vi "_LOharmonic.vi"(0 "Bias_LO_equip":T5={"Node address"=19, "CAN Interface"="CAN0", "Cartridge band"=10, "Slave Node in"={"Address"=19, "Serial Number"=[16, -88, -112, 75, 1, 8, 0, 24]}, "ObjHandle out"=19, "POL"=0, "sb"=1, "GPIB_SM (SIS S,V)"="24", "GPIB_DMM (SIS I)"="22", "GPIB_SM (MAG I) "="25", "GPIB_SG(LO)"="19", "GPIB_PW (PAMP) "="6", "GPIB_TMP1(8ch)"="12", "GPIB_TMP2(2ch)  "="13", "WCA_avg"=10, "Rsen"=10.0, "BiasModule"=1, "LOModule "=2, "WCA_LO_FREQ_SET"={"YTO Low freq. [GHz]"=14.66, "YTO High freq. [GHz]"=17.5, "Kvco"=1, "Lock Pol."=0, "SET LO FREQ"=88.77778, "Multiplier"=6.0, "YTO (HEX)"=197, "YTO ( FREQ)"=14.796625, "NULL PLL INTEGRATOR"=FALSE}, "Res for"=0} {"Res for" items=["none", "series res", "parallel res"]; "WCA_LO_FREQ_SET"."YTO ( FREQ)" min=25 max=150 step=0.0001 format="%.3f"; "WCA_LO_FREQ_SET"."Multiplier" min=3 max=6 step=3; "WCA_LO_FREQ_SET"."SET LO FREQ" min=25 max=150 step=0.0001 format="%.3f"; "WCA_LO_FREQ_SET"."Lock Pol." items=["Lower", "Upper"]; "WCA_LO_FREQ_SET"."Kvco" items=["7.5MHz/V", "15MHz/V"]; "WCA_LO_FREQ_SET"."YTO High freq. [GHz]" format="%.3f"; "WCA_LO_FREQ_SET"."YTO Low freq. [GHz]" format="%.3f"; "LOModule" items=["Manual Gunn+PAMP"=0, "PLL GUNN+PAMP"=5, "B10Lab LO"=1, "WCA LO"=2, ""=3, "YIG発信器"=4, "none"=99]; "BiasModule" items=["B10Lab Bias"=0, "WCA BiasModule"=1, "none"=99]; "Slave Node in"."Serial Number" format="%.0x"; "Slave Node in"."Address" format="%.0x"; "Cartridge band" max=10 step=1; "Node address" format="%.0x"}, 1 "Control":T9={"GPIB_ATT"="28", "6501Dev#"=1, "GPIB_SP"="18", "GPIB_PM"="13", "GPIB_DSA"="11", "GPIB_DMM (TPD)"="23", "GPIB_MPI"="COM3", "mortor設定"=[{"Axis"=0, "ID"=0, "HIspeed"=200.0, "LOspeed"=100.0, "ACCEL(ms)"=100.0, "Sratio"=50.0, "フリーラン\n"=FALSE, "文字列"="DSB HOT/COLD"}, {"Axis"=1, "ID"=0, "HIspeed"=4.0, "LOspeed"=4.0, "ACCEL(ms)"=100.0, "Sratio"=50.0, "フリーラン\n"=TRUE, "文字列"="SubMM Att"}, {"Axis"=0, "ID"=0, "HIspeed"=200.0, "LOspeed"=100.0, "ACCEL(ms)"=100.0, "Sratio"=50.0, "フリーラン\n"=FALSE, "文字列"="MPI Port1"}, {"Axis"=1, "ID"=0, "HIspeed"=200.0, "LOspeed"=100.0, "ACCEL(ms)"=100.0, "Sratio"=50.0, "フリーラン\n"=FALSE, "文字列"="MPI Port2"}, {"Axis"=1, "ID"=0, "HIspeed"=200.0, "LOspeed"=100.0, "ACCEL(ms)"=100.0, "Sratio"=50.0, "フリーラン\n"=TRUE, "文字列"="gainComp"}], "DATAパス"=path "C:/Documents and Settings/band10/デスクトップ/data/cartridge/CCA03/CCA-03-13/110831_etc", "mixer param file "=path "C:/Users/band10/Desktop/data/cartridge/CCA02/111107_CCA02-08_mixparam.csv", "comment"="xttest", "ColdCarts"="003601", "Th"=299.0, "Tc"=77.0, "Set_SIS_volt"=2.25, "Offset"=0.0, "control"=0, "FreqLO"=938.25, "Set_Mag_Cur"=13.664233576642335, "MPI offset(mm)"=23.152, "HOT/COLD"=0} {"HOT/COLD" items=["DSB", "SBR (Cart.)", "GainComp", "SBR (MIX)"]; "control" items=["CLOSE LOOP", "OPEN LOOP", "Not Control"]}, 2 "LOhharmonic":T8={"save"=FALSE, "file_name"="xtk_799.00_120_xttest.csv", "LO start"=794.0, "LO stop"=834.0, "LO step"=8.0, "IF"=5.0, "8th 10th"=FALSE}, 3 "PAV配列":cluster{"VD":dbl, "VG ":dbl, "文字列":string}[](array[cluster])=[{"VD"=0.0, "VG "=-0.04, "文字列"="WCA P0"}, {"VD"=0.0, "VG "=-0.04, "文字列"="WCA P1"}, {"VD"=1.75, "VG "=2.1, "文字列"="B10 PAMP"}] {"VG" min=-1.0 max=4.0; "VD" min=0.0 max=2.5}, 4 "_LO_P_OPT":T4={"範囲配列"=[{"Start"=1.0, "Stop"=3.5, "Step"=0.01, "ｂｙ"="NEL VG"}, {"Start"=40.0, "Stop"=75.0, "Step"=1.0, "ｂｙ"="Motor"}, {"Start"=1.0, "Stop"=2.5, "Step"=0.1, "ｂｙ"="WCA VD"}], "Optimize"=0, "file_name"="LP_914.0_Tmin_100519.csv", "Save?"=FALSE, "measure"=2, "current(uA)"=60.0, "wait(ms)"=0, "IFfrq(GHz)"=8.0, "aveg"=10, "SISparam option"=2} {"SISparam option" items=["Volt and Current", "Volt only"]; "measure" items=["Pmax (only HOT)", "Tmin (HOT/COLD)", "C current"]; "Optimize" items=["Sweep", "黄金分割"]; "範囲配列"."Step" format="%.2f"; "範囲配列"."Stop" format="%.2f"; "範囲配列"."Start" format="%.2f"}) -> (7 "LOPopt":string="LOPt,834.00,2.03,2.02,27.31,0.00,0.00,0.00,0.31,,WCA,0.008698,3.219604,-0.035706,  3.273315,362.594604,-0.035858,")   [LabVIEW 2017]
uses:
  <vilib>/express/express arith-compare/Formula/XNode/ExpressFormulaBlockNode.xnode
panel:
  in  "LO_misc":T1={"LO FRQ(GHz)"=898.875, "LO multi "=9.0, "LocK?"=TRUE, "LO REF multi"=3.0, "wait (ms)"=100.0, "SG Pow Min (dBm)"=0.0, "SG Pow Max (dBm)"=20.0, "SG Pow Step (dBm)"=0.2, "SGPow OPT? "=TRUE, "SG set frq"=29.60259259259259, "SG set pow"=0.0}
  out "結果":string="794.000000,799.000000,5.000009,-9.796000,  893.250000,5.000006,-43.635000,  33.839000, LOPt,794.00,2.40,1.97,26.51,0.00,0.00,0.00,0.49,,WCA,0.008545,5.584717,-0.035858,  3.854065,400.955200,-0.036011, ,LOPt,893.25,2.33,2.16,27.34,0.00,0.00,0.00,0.34,,WCA,0.008392,2.838135,-0.035553,  3.744507,317.977905,-0.036316, \n802.000000,807.000000,4.999982,-9.118000,  902.250000,4.999982,-49.373000,  40.255000, LOPt,802.00,2.04,2.02,26.22,0.00,0.00,0.00,0.78,,WCA,0.008545,3.829956,-0.035706,  3.288879,368.423462,-0.036011, ,LOPt,902.25,2.47,2.07,26.05,0.00,0.00,0.00,0.95,,WCA,0.008545,2.761841,-0.035706,  3.962097,323.913574,-0.035858, \n810.000000,815.000000,5.000036,-9.253000,  911.250000,5.000036,-42.998000,  33.745000, LOPt,810.00,2.26,2.07,25.96,0.00,0.00,0.00,1.04,,WCA,0.008698,3.234863,-0.035858,  3.635712,396.102905,-0.036011, ,LOPt,911.25,2.47,2.13,25.31,0.00,0.00,0.00,1.69,,WCA,0.008545,2.593994,-0.035858,  3.961945,320.861816,-0.036163, \n818.000000,823.000000,5.000036,-10.017000,  920.250000,5.000036,-58.467000,  48.450000, LOPt,818.00,2.33,2.02,27.34,0.00,0.00,0.00,0.34,,WCA,0.008698,3.250122,-0.035400,  3.744812,403.976440,-0.035858, ,LOPt,920.25,1.82,2.13,27.02,0.00,0.00,0.00,0.02,,WCA,0.008392,2.105713,-0.035706,  2.941284,269.073486,-0.036163, \n826.000000,831.000000,5.000009,-9.863000,  929.250000,5.000012,-49.319000,  39.456000, LOPt,826.00,2.26,2.07,26.90,0.00,0.00,0.00,0.10,,WCA,0.008545,3.021240,-0.035400,  3.635559,392.822266,-0.036163, ,LOPt,929.25,1.90,2.16,26.92,0.00,0.00,0.00,0.08,,WCA,0.008545,1.922607,-0.035706,  3.051300,262.527466,-0.036469, \n834.000000,839.000000,5.000009,-13.918000,  938.250000,5.000012,-36.992000,  23.074000, LOPt,834.00,2.03,2.02,27.31,0.00,0.00,0.00,0.31,,WCA,0.008698,3.219604,-0.035706,  3.273315,362.594604,-0.035858, ,LOPt,938.25,2.33,2.17,27.53,0.00,0.00,0.00,0.53,,WCA,0.008545,1.785278,-0.035706,  3.743896,280.242920,-0.036011, \n"
  out "XYグラフ":cluster{dbl[], dbl[]}[](graph)=[{[794.0, 802.0, 810.0, 818.0, 826.0, 834.0], [-9.796, -9.118, -9.253, -10.017, -9.863, -13.918]}, {[794.0, 802.0, 810.0, 818.0, 826.0, 834.0], [-43.635, -49.373, -42.998, -58.467, -49.319, -36.992]}]
  out "HLOPopt":string="LOPt,938.25,2.33,2.17,27.53,0.00,0.00,0.00,0.53,,WCA,0.008545,1.785278,-0.035706,  3.743896,280.242920,-0.036011,"
  out "H IF":dbl=5.000012338 format="%#_6p"
  out "H LO":dbl=938.25 format="%#_6p"
  out "RF":dbl=839.0 format="%#_6p"
  in  "SP_set":T2={"start(GHz)"=3.5, "stop(GHz) "=12.5, "BW(MHz)"=0.0001, "VBW(Hz)"=30.0, "ref(dBm)"=0.0, "log(dB)"=15.0, "AVEG"=30, "AVEG ON/OFF"=FALSE, "Auto Align ON/OFF"=FALSE, "GPIB"="18", "point"=801}
  in  "IFBOX":T3={" Output"=1, "YIG Fc(GHz)"=4.0, " Filter"=3, "Input"=1} {"Input" items=["1:Pol 0"=1, "2:Pol 1"=2, "3:dummy"=3, "4:NoiseSource"=4]; "Filter" items=["1:YIG"=1, "2:direct"=2, "3:4-12BPF"=3, "4:direct 4-12BPF"=4]; "Output" items=["1:Speana"=1, "2:PowerMeter"=2, "3:dummy"=3, "4:TPD"=4]}
  in  "RF":T6={"RF(GHz)"=800.0, "mm_multi(4or6)"=6.0, "SGPOUT(dBm)"=10.0, "SGGPIB"="29", "PAMP GPIB"="6", "VD (V)"=1.7, "VG (V)"=2.2, "multi (V)"=8.0} {"multi (V)" min=0.0 max=15.0 step=0.5; "VG (V)" min=0.0 max=4.0 step=0.1; "VD (V)" min=0.0 max=1.85 step=0.1}
  out "IF":dbl=5.000009331 format="%#_6p"
  out "H IF Pow":dbl=-36.992 format="%#_6p"
  out "IF Pow":dbl=-13.918 format="%#_6p"
  out "LO":dbl=834.0 format="%#_6p"
  in  "SIS_Deflux_heater":T7={"ON開始時間（mｓ）"=3000.0, "ON継続時間（mｓ）"=1000.0, "測定終了時間（mｓ）"=60000.0, "SIS Volt（mV)"=0.5, "GPIB_PW (SISHeater) "="3", "SAVE"=TRUE}
  out "初期時間（s）":dbl=3379641043.615625
  # "LO freq. [GHz]"
  # "YTO LOW\n/High Freq."
  # "ZERO Intgrtr"
  # "Node Address"
  # "Serial Number"
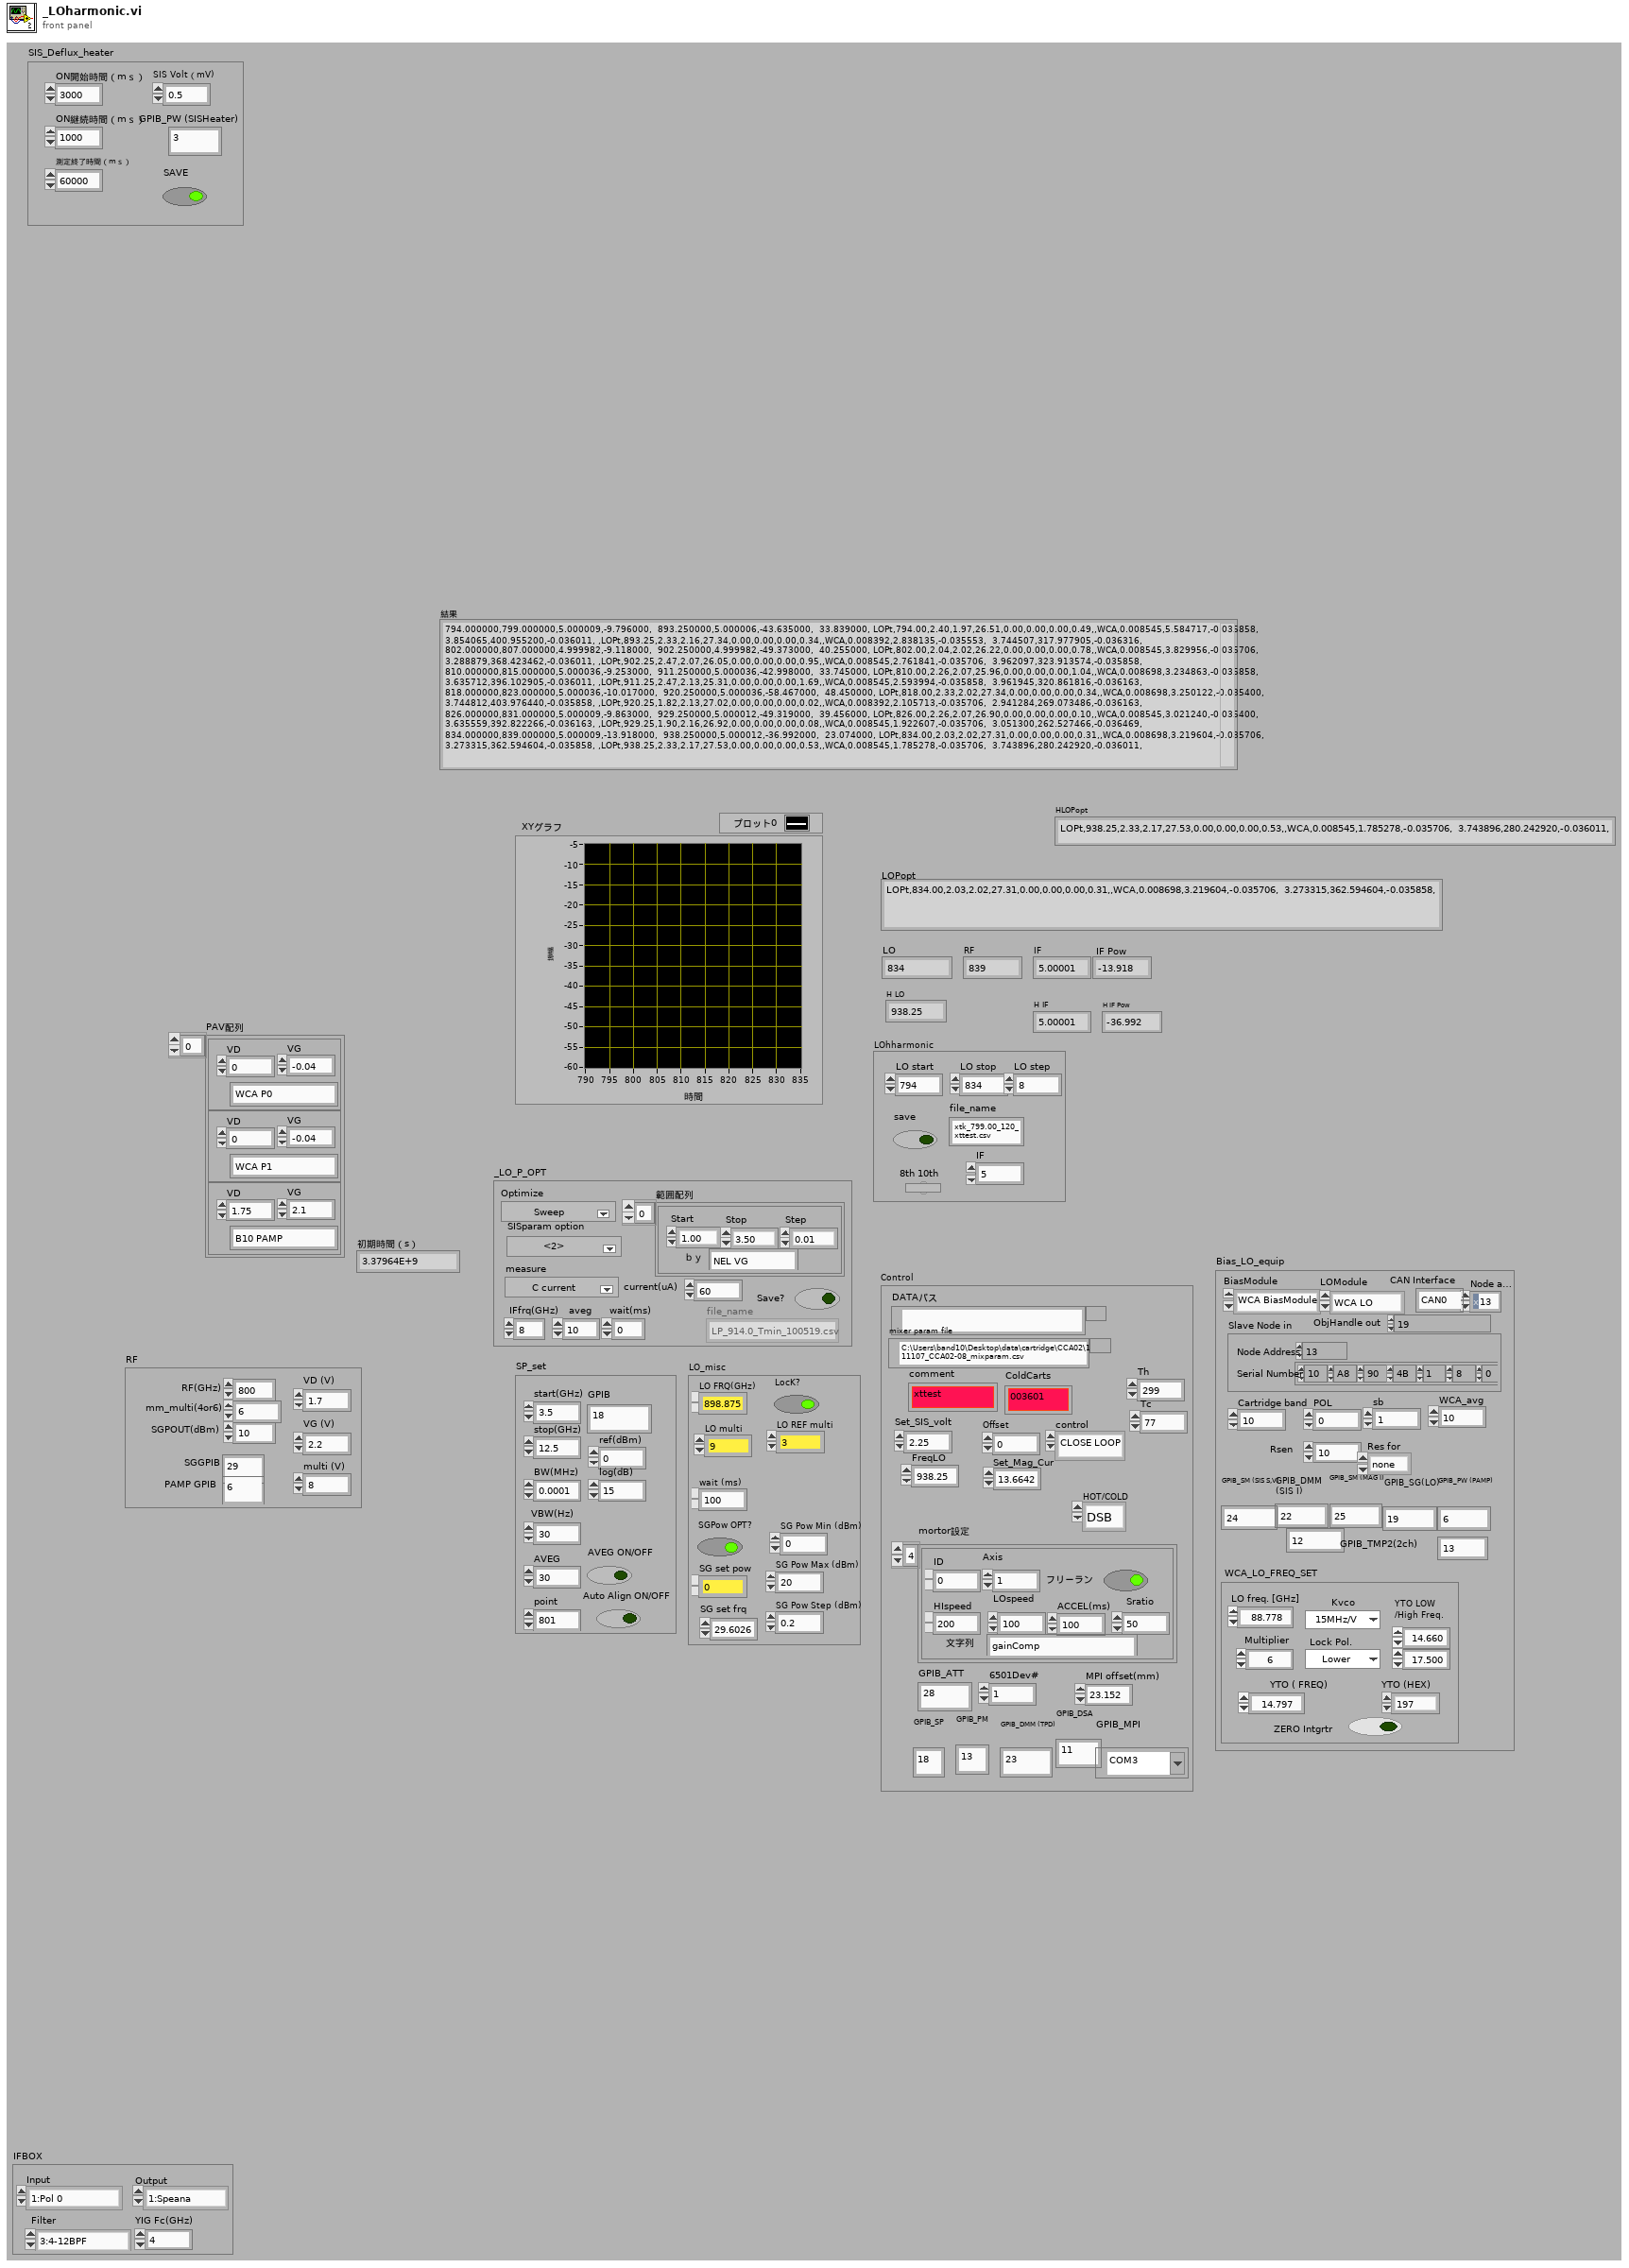
[diagram p1: front panel]
types:
  T1 = cluster{"LO FRQ(GHz)":dbl, "LO multi ":dbl, "LocK?":bool, "LO REF multi":dbl, "wait (ms)":dbl, "SG Pow Min (dBm)":dbl, "SG Pow Max (dBm)":dbl, "SG Pow Step (dBm)":dbl, "SGPow OPT? ":bool, "SG set frq":dbl, "SG set pow":dbl}
  T2 = cluster{"start(GHz)":dbl, "stop(GHz) ":dbl, "BW(MHz)":dbl, "VBW(Hz)":dbl, "ref(dBm)":dbl, "log(dB)":dbl, "AVEG":i16, "AVEG ON/OFF":bool, "Auto Align ON/OFF":bool, "GPIB":string, "point":i16}
  T3 = cluster{" Output":u16, "YIG Fc(GHz)":dbl, " Filter":u16, "Input":u16}
  T4 = cluster{"範囲配列":cluster{"Start":dbl, "Stop":dbl, "Step":dbl, "ｂｙ":string}[], "Optimize":u16, "file_name":string, "Save?":bool, "measure":u16, "current(uA)":dbl, "wait(ms)":i32, "IFfrq(GHz)":dbl, "aveg":i32, "SISparam option":u16}
  T5 = cluster{"Node address":u16, "CAN Interface":string, "Cartridge band":u32, "Slave Node in":cluster{"Address":i16, "Serial Number":i8[]}, "ObjHandle out":u32, "POL":u32, "sb":u32, "GPIB_SM (SIS S,V)":string, "GPIB_DMM (SIS I)":string, "GPIB_SM (MAG I) ":string, "GPIB_SG(LO)":string, "GPIB_PW (PAMP) ":string, "GPIB_TMP1(8ch)":string, "GPIB_TMP2(2ch)  ":string, "WCA_avg":i32, "Rsen":dbl, "BiasModule":u16, "LOModule ":u16, "WCA_LO_FREQ_SET":cluster{"YTO Low freq. [GHz]":sgl, "YTO High freq. [GHz]":sgl, "Kvco":u16, "Lock Pol.":u16, "SET LO FREQ":sgl, "Multiplier":sgl, "YTO (HEX)":u16, "YTO ( FREQ)":sgl, "NULL PLL INTEGRATOR":bool}, "Res for":u16}
  T6 = cluster{"RF(GHz)":dbl, "mm_multi(4or6)":dbl, "SGPOUT(dBm)":dbl, "SGGPIB":string, "PAMP GPIB":string, "VD (V)":dbl, "VG (V)":dbl, "multi (V)":dbl}
  T7 = cluster{"ON開始時間（mｓ）":dbl, "ON継続時間（mｓ）":dbl, "測定終了時間（mｓ）":dbl, "SIS Volt（mV)":dbl, "GPIB_PW (SISHeater) ":string, "SAVE":bool}
  T8 = cluster{"save":bool, "file_name":string, "LO start":dbl, "LO stop":dbl, "LO step":dbl, "IF":dbl, "8th 10th":bool}
  T9 = cluster{"GPIB_ATT":string, "6501Dev#":i16, "GPIB_SP":string, "GPIB_PM":string, "GPIB_DSA":string, "GPIB_DMM (TPD)":string, "GPIB_MPI":refnum<visa-resource-name>, "mortor設定":cluster{"Axis":i16, "ID":i16, "HIspeed":dbl, "LOspeed":dbl, "ACCEL(ms)":dbl, "Sratio":dbl, "フリーラン\n":bool, "文字列":string}[], "DATAパス":path, "mixer param file ":path, "comment":string, "ColdCarts":string, "Th":dbl, "Tc":dbl, "Set_SIS_volt":dbl, "Offset":dbl, "control":u16, "FreqLO":dbl, "Set_Mag_Cur":dbl, "MPI offset(mm)":dbl, "HOT/COLD":u16}
  T10 = cluster{"GPIB_ATT":string, "6501Dev#":i16, "GPIB_SP":string, "GPIB_PM":string, "GPIB_DSA":string, "GPIB_DMM (TPD)":string, "GPIB_MPI":string, "mortor設定":cluster{"Axis":i16, "ID":i16, "HIspeed":dbl, "LOspeed":dbl, "ACCEL(ms)":dbl, "Sratio":dbl, "フリーラン\n":bool, "文字列":string}[], "DATAパス":path, "DBパス ":path, "comment":string, "ColdCarts":string, "Th":dbl, "Tc":dbl, "Set_SIS_volt":dbl, "Offset":dbl, "control":u16, "FreqLO":dbl, "Set_Mag_Cur":dbl, "MPI offset(mm)":dbl, "HOT/COLD":u16}
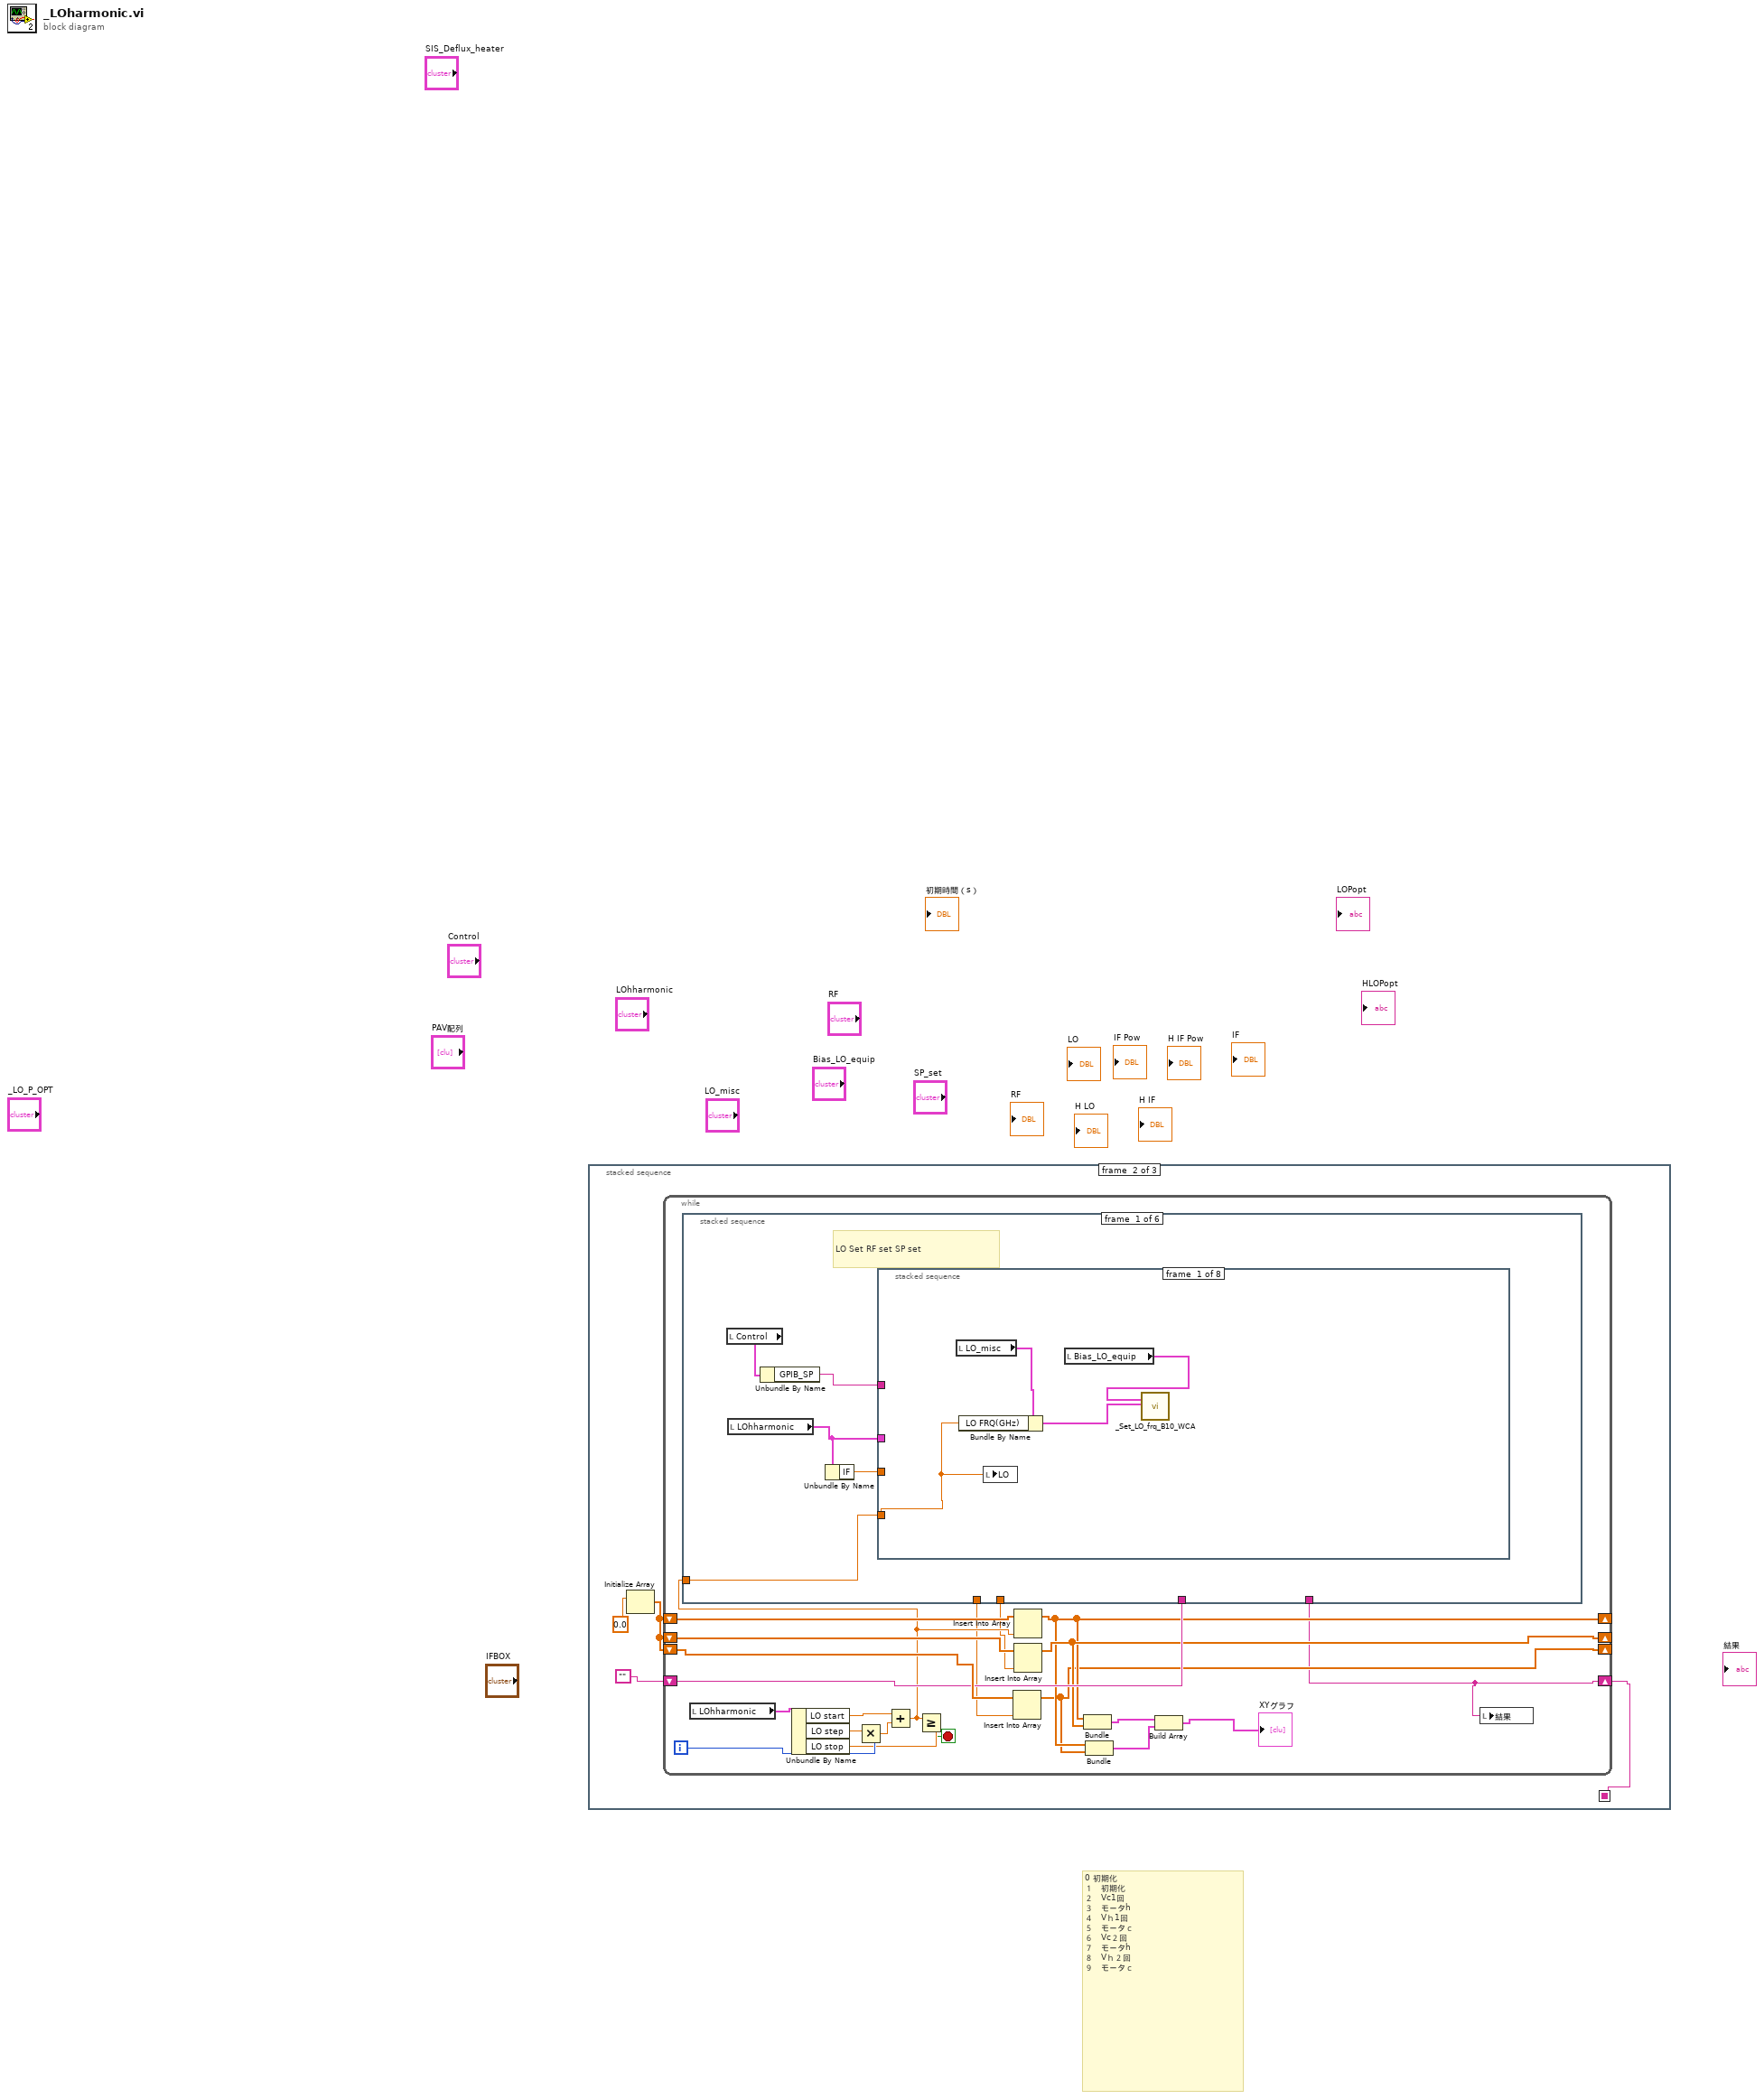
[diagram p0: block diagram]
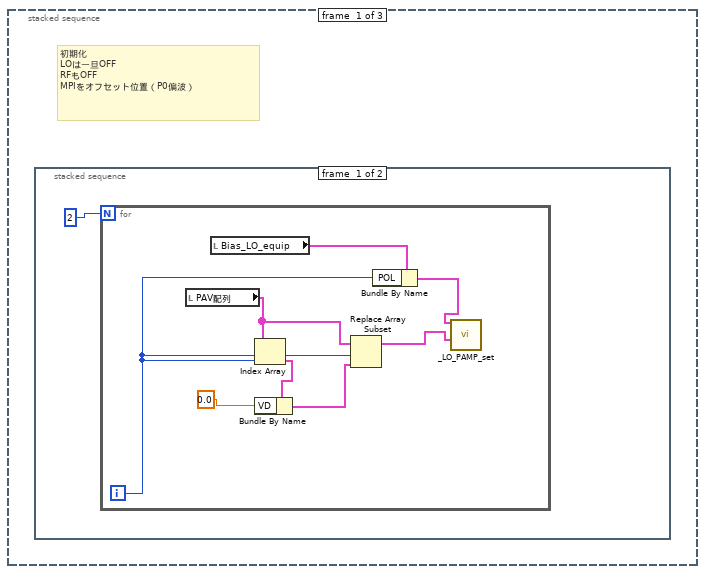
[diagram p2: hidden frame]
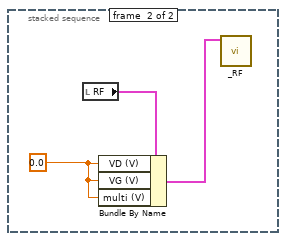
[diagram p3: hidden frame]
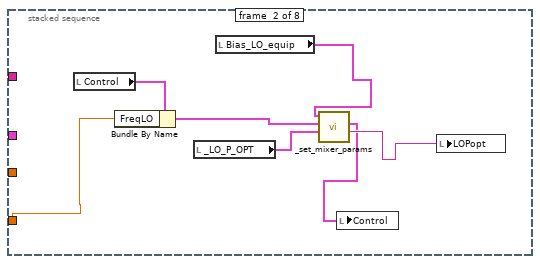
[diagram p4: hidden frame]
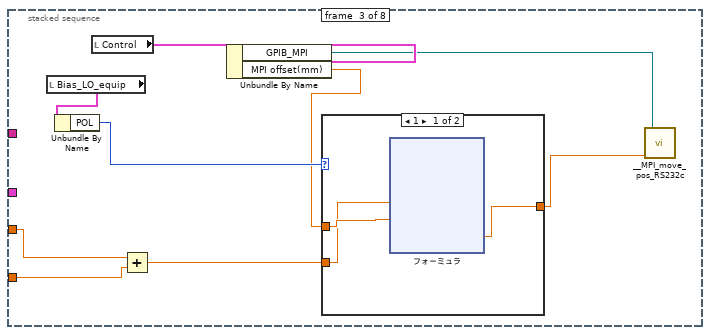
[diagram p5: hidden frame]
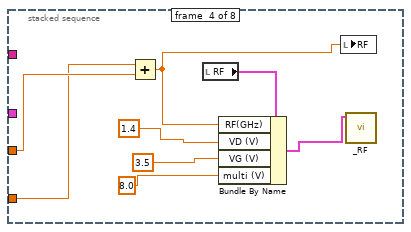
[diagram p7: hidden frame]
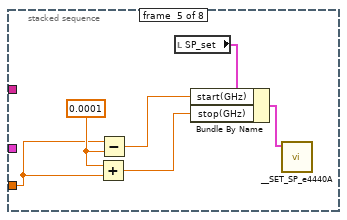
[diagram p8: hidden frame]
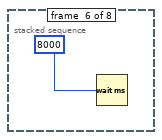
[diagram p9: hidden frame]
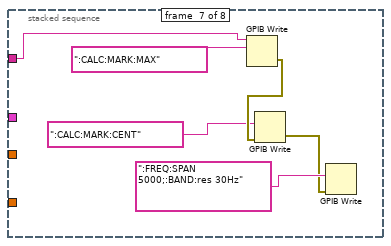
[diagram p10: hidden frame]
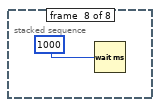
[diagram p11: hidden frame]
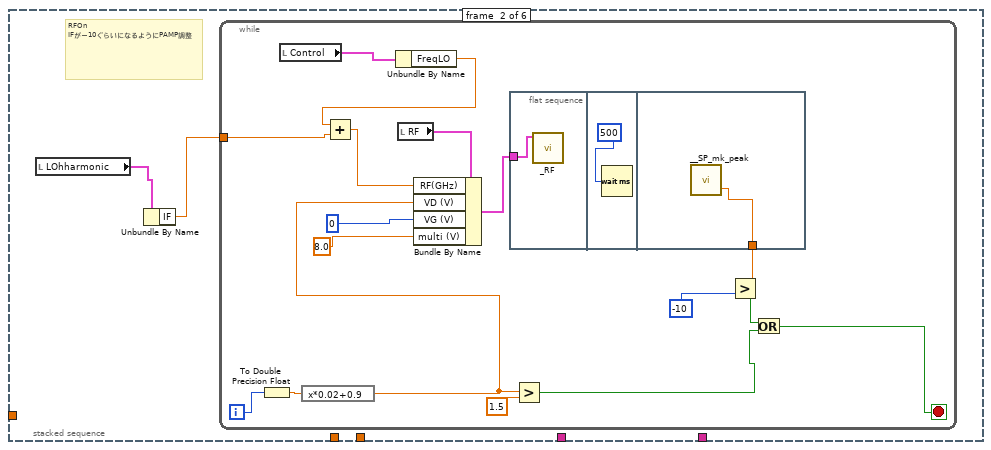
[diagram p12: hidden frame]
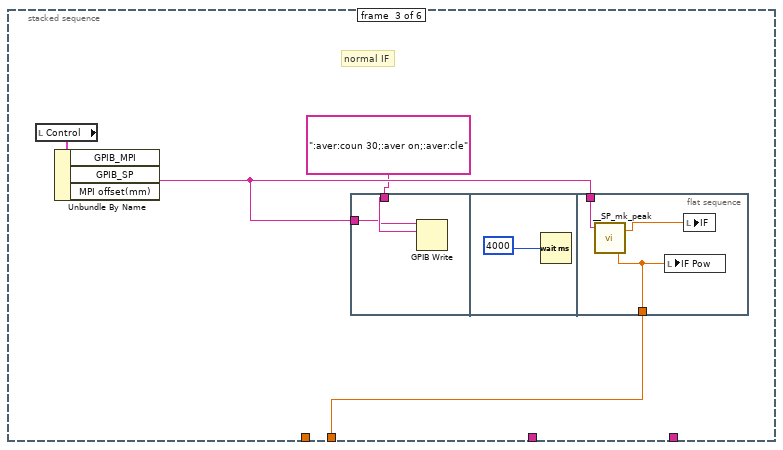
[diagram p13: hidden frame]
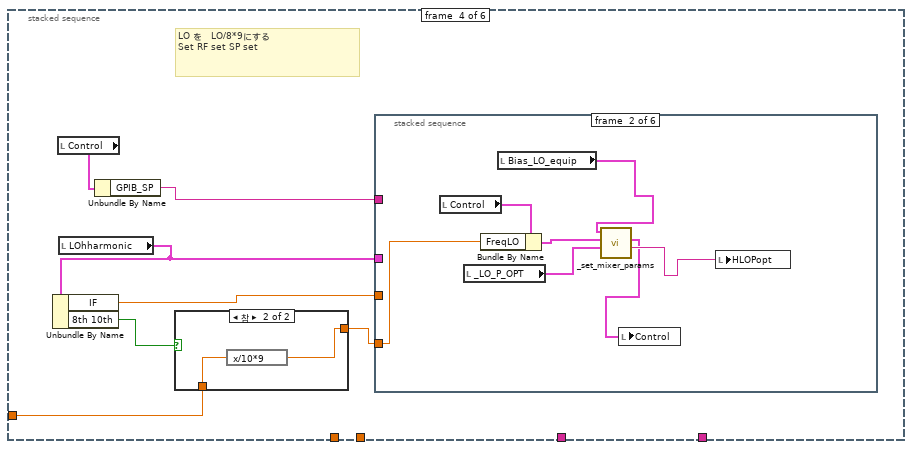
[diagram p14: hidden frame]
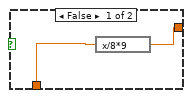
[diagram p15: hidden frame]
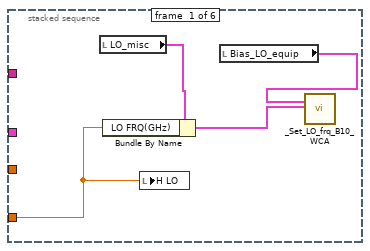
[diagram p16: hidden frame]
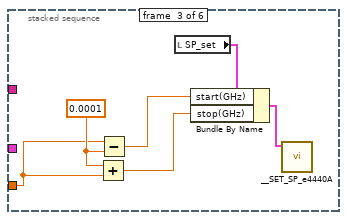
[diagram p17: hidden frame]
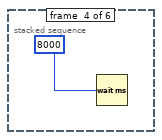
[diagram p18: hidden frame]
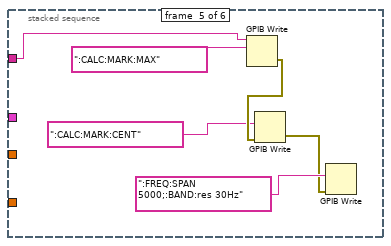
[diagram p19: hidden frame]
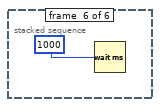
[diagram p20: hidden frame]
diagram:
  # "0 初期化\n１　初期化\n２　Vc1回\n３　モータh\n４　Vｈ1回\n５　モータｃ\n６　Vc２回\n７　モータh\n８　Vｈ２回\n９　モータｃ"
  n1 = stacked-sequence {
    seq-local: [_ w13 _] -> [_ _ w190]
    frame #0 {
      # "初期化\nLOは一旦OFF\nRFもOFF\nMPIをオフセット位置（P0偏波）"
      n2 = stacked-sequence {
        frame #0 {
          n3 = for {
            N: 2 -> [_]
            i -> [w2]
            n4 = local read "PAV配列"() -> (w5:cluster{"VD":dbl, "VG ":dbl, "文字列":string}[])
            n5 = local read "Bias_LO_equip"() -> (w4:T5)
            n6 = Index Array(array=w5, index=w2) -> (element=w8:cluster{"VD":dbl, "VG ":dbl, "文字列":string})
            n7 = Bundle By Name(cluster=w8, "VD"=0.0) -> (w9:cluster{"VD":dbl, "VG ":dbl, "文字列":string})
            n8 = Replace Array Subset(array=w5, new element=w9, index=w2) -> (w7:cluster{"VD":dbl, "VG ":dbl, "文字列":string}[])
            n9 = Bundle By Name(cluster=w4, "POL"=w2) -> (w3:T5)
            n10 = call "_LO_PAMP_set.vi"("PAV配列"=w7, "Bias_LO_equip"=w3) -> ()  [unwired: 10 in]
          }
        }
        frame #1 {
          w11 = 0.0
          n11 = local read "RF"() -> (w12:T6)
          n12 = Bundle By Name(cluster=w12, "VD (V)"=w11, "VG (V)"=w11, "multi (V)"=w11) -> (w10:T6)
          n13 = call "_RF.vi"("RF"=w10) -> ()  [unwired: 11 in]
        }
      }
    }
    frame #1 {
      n14 = Initialize Array(0.0) -> (w15:dbl[])  [unwired: 1 in]
      n15 = while {
        shift-right: [w25] -> _
        shift-left: w15 -> [w30]
        shift-right: [w26] -> _
        shift-left: w15 -> [w29]
        shift-right: [w24] -> _
        shift-left: w15 -> [w28]
        shift-right: [w20] -> w13
        shift-left: "" -> [w27]
        i -> [w35]
        stop <- w31 stop-if-true
        n16 = local read "LOhharmonic"() -> (w37:T8)
        n17 = Unbundle By Name(w37) -> ("LO start"=w34:dbl, "LO step"=w36:dbl, "LO stop"=w32:dbl)
        n18 = Multiply(x=w36, y=w35) -> (x*y=w33:dbl)
        n19 = Add(x=w34, y=w33) -> (x+y=w19:dbl)
        n20 = stacked-sequence {
          tunnel: w19 -> [w42 _ _ w133 _ _]
          tunnel: w27 -> [_ _ _ _ _ w188]
          tunnel: [_ _ _ _ _ w187] -> w20
          tunnel: [_ _ w121 _ _ _] -> w18
          tunnel: [_ _ _ _ w167 _] -> w17
          frame #0 {
            # "LO Set RF set SP set"
            n21 = local read "Control"() -> (w41:T9)
            n22 = local read "LOhharmonic"() -> (w39:T8)
            n23 = Unbundle By Name(w41) -> ("GPIB_SP"=w40:string)
            n24 = Unbundle By Name(w39) -> ("IF"=w38:dbl)
            n25 = stacked-sequence {
              tunnel: w42 -> [w43 w49 w55 w77 _ _ _ _]
              tunnel: w40 -> [_ _ _ _ _ _ w96 _]
              tunnel: w39 -> [_ _ _ _ _ _ _ _]
              tunnel: w38 -> [_ _ w56 w79 w85 _ _ _]
              frame #0 {
                n26 = local read "LO_misc"() -> (w44:T1)
                n27 = Bundle By Name(cluster=w44, "LO FRQ(GHz)"=w43) -> (w45:T1)
                n28 = local write "LO"(w43) -> ()
                n29 = local read "Bias_LO_equip"() -> (w46:T5)
                n30 = call "_Set_LO_frq_B10_WCA.vi"("Bias_LO_equip"=w46, "LO_misc"=w45) -> ()  [unwired: 15 in, 3 out]
              }
              frame #1 {
                n31 = local read "Control"() -> (w50:T9)
                n32 = Bundle By Name(cluster=w50, "FreqLO"=w49) -> (w48:T9)
                n33 = local read "_LO_P_OPT"() -> (w53:T4)
                n34 = local read "Bias_LO_equip"() -> (w51:T5)
                n35 = call "_set_mixer_params.vi"("_LO_P_OPT"=w53, "Control"=w48, "Bias_LO_equip"=w51) -> ("文字列"=w52:string, "Control 2"=w47:T10)  [unwired: 6 in, 1 out]
                n36 = local write "Control"(w47) -> ()
                n37 = local write "LOPopt"(w52) -> ()
              }
              frame #2 {
                n38 = local read "Bias_LO_equip"() -> (w62:T5)
                n39 = Unbundle By Name(w62) -> ("POL"=w61:u32)
                n40 = local read "Control"() -> (w60:T9)
                n41 = Add(x=w56, y=w55) -> (x+y=w54:dbl)
                n42 = Unbundle By Name(w60) -> ("GPIB_MPI"=w59:refnum<visa-resource-name>, "MPI offset(mm)"=w57:dbl)
                n43 = case shown="1" w61 {
                  tunnel: [w63 w76] -> w58
                  tunnel: w57 -> [w65 w76]
                  tunnel: w54 -> [w64 _]
                  frame 1 {
                    n44 = xnode "フォーミュラ"("RF"=w64, "offset"=w65) -> ("結果"=w63:dbl)  [unwired: 1 in, 1 out]
                  }
                  frame 0, Default {
                  }
                }
                n45 = call "__MPI_move_pos_RS232c.vi"("pos"=w58, "VISAリソース名"=w59) -> ()  [unwired: 5 in, 1 out]
              }
              frame #3 {
                n46 = Add(x=w77, y=w79) -> (x+y=w78:dbl)
                n47 = local read "RF"() -> (w84:T6)
                n48 = Bundle By Name(cluster=w84, "RF(GHz)"=w78, "VD (V)"=1.4, "VG (V)"=3.5, "multi (V)"=8.0) -> (w80:T6)
                n49 = local write "RF"(w78) -> ()
                n50 = call "_RF.vi"("RF"=w80) -> ()  [unwired: 11 in]
              }
              frame #4 {
                w88 = 0.0001
                n51 = Add(x=w88, y=w85) -> (x+y=w86:dbl)
                n52 = Subtract(x=w85, y=w88) -> (x-y=w87:dbl)
                n53 = local read "SP_set"() -> (w89:T2)
                n54 = Bundle By Name(cluster=w89, "start(GHz)"=w87, "stop(GHz)"=w86) -> (w90:T2)
                n55 = call "__SET_SP_e4440A.vi"("SP"=w90) -> ()  [unwired: 7 in]
              }
              frame #5 {
                n56 = Wait (ms)(milliseconds to wait=8000) -> ()  [unwired: 1 out]
              }
              frame #6 {
                n57 = GPIB Write(0:w96, 1:":CALC:MARK:MAX") -> (6:w95:errorcluster)  [unwired: 3 in, 1 out]
                n58 = GPIB Write(1:":CALC:MARK:CENT", 3:w95) -> (6:w92:errorcluster)  [unwired: 3 in, 1 out]
                n59 = GPIB Write(1:":FREQ:SPAN 5000;:BAND:res 30Hz", 3:w92) -> ()  [unwired: 3 in, 2 out]
              }
              frame #7 {
                n60 = Wait (ms)(milliseconds to wait=1000) -> ()  [unwired: 1 out]
              }
            }
          }
          frame #1 {
            # "RFOn\nIFがー10ぐらいになるようにPAMP調整"
            n61 = local read "LOhharmonic"() -> (w100:T8)
            n62 = Unbundle By Name(w100) -> ("IF"=w99:dbl)
            n63 = while {
              tunnel: w99 -> [w101]
              i -> [w117]
              stop <- w105 stop-if-true
              n64 = To Double Precision Float(number=w117) -> (double precision float=w116:dbl)
              n65 = local read "Control"() -> (w104:T9)
              n66 = expression code="x*0.02+0.9"(w116) -> (w112:dbl)
              n67 = Unbundle By Name(w104) -> ("FreqLO"=w102:dbl)
              n68 = Add(x=w102, y=w101) -> (x+y=w103:dbl)
              n69 = local read "RF"() -> (w114:T6)
              n70 = Bundle By Name(cluster=w114, "RF(GHz)"=w103, "VD (V)"=w112, "VG (V)"=0, "multi (V)"=8.0) -> (w113:T6)
              n71 = flat-sequence {
                tunnel: w113 -> [w118]
                tunnel: [w120] -> w109
                frame #0 {
                  n72 = call "_RF.vi"("RF"=w118) -> ()  [unwired: 11 in]
                }
                frame #1 {
                  n73 = Wait (ms)(milliseconds to wait=500) -> ()  [unwired: 1 out]
                }
                frame #2 {
                  n74 = call "__SP_mk_peak.vi"() -> ("pow out"=w120:dbl)  [unwired: 3 in, 1 out]
                }
              }
              n75 = Greater?(x=w112, y=1.5) -> (0:w106:bool)
              n76 = Greater?(x=w109, y=-10) -> (0:w107:bool)
              n77 = Or(x=w107, y=w106) -> (x .or. y?=w105:bool)
            }
          }
          frame #2 {
            # "normal IF"
            n78 = local read "Control"() -> (w124:T9)
            n79 = Unbundle By Name(w124) -> ("GPIB_SP"=w123:string)  [unwired: 2 out]
            n80 = flat-sequence {
              tunnel: ":aver:coun 30;:aver on;:aver:cle" -> [w126]
              tunnel: w123 -> [w125]
              tunnel: w123 -> [w130]
              tunnel: [w128] -> w121
              frame #0 {
                n81 = GPIB Write(0:w125, 1:w126) -> ()  [unwired: 3 in, 2 out]
              }
              frame #1 {
                n82 = Wait (ms)(milliseconds to wait=4000) -> ()  [unwired: 1 out]
              }
              frame #2 {
                n83 = call "__SP_mk_peak.vi"("GIPB番号"=w130) -> ("pow out"=w128:dbl, "Freq out"=w129:dbl)  [unwired: 2 in]
                n84 = local write "IF Pow"(w128) -> ()
                n85 = local write "IF"(w129) -> ()
              }
            }
          }
          frame #3 {
            # "LO を　LO/8*9にする\nSet RF set SP set"
            n86 = local read "Control"() -> (w137:T9)
            n87 = local read "LOhharmonic"() -> (w135:T8)
            n88 = Unbundle By Name(w135) -> ("IF"=w134:dbl, "8th 10th"=w131:bool)
            n89 = Unbundle By Name(w137) -> ("GPIB_SP"=w136:string)
            n90 = case shown="참" w131 {
              tunnel: w133 -> [w139 w141]
              tunnel: [w138 w140] -> w132
              frame False {
                n91 = expression code="x/8*9"(w139) -> (w138:dbl)
              }
              frame True {
                n92 = expression code="x/10*9"(w141) -> (w140:dbl)
              }
            }
            n93 = stacked-sequence {
              tunnel: w132 -> [w142 w146 _ _ _ _]
              tunnel: w136 -> [_ _ _ _ w164 _]
              tunnel: w135 -> [_ _ _ _ _ _]
              tunnel: w134 -> [_ _ w153 _ _ _]
              frame #0 {
                n94 = local read "LO_misc"() -> (w143:T1)
                n95 = Bundle By Name(cluster=w143, "LO FRQ(GHz)"=w142) -> (w144:T1)
                n96 = local write "H LO"(w142) -> ()
                n97 = local read "Bias_LO_equip"() -> (w145:T5)
                n98 = call "_Set_LO_frq_B10_WCA.vi"("Bias_LO_equip"=w145, "LO_misc"=w144) -> ()  [unwired: 15 in, 3 out]
              }
              frame #1 {
                n99 = local read "Control"() -> (w149:T9)
                n100 = local read "_LO_P_OPT"() -> (w152:T4)
                n101 = Bundle By Name(cluster=w149, "FreqLO"=w146) -> (w148:T9)
                n102 = local read "Bias_LO_equip"() -> (w150:T5)
                n103 = call "_set_mixer_params.vi"("_LO_P_OPT"=w152, "Control"=w148, "Bias_LO_equip"=w150) -> ("文字列"=w151:string, "Control 2"=w147:T10)  [unwired: 6 in, 1 out]
                n104 = local write "Control"(w147) -> ()
                n105 = local write "HLOPopt"(w151) -> ()
              }
              frame #2 {
                w156 = 0.0001
                n106 = Add(x=w156, y=w153) -> (x+y=w154:dbl)
                n107 = Subtract(x=w153, y=w156) -> (x-y=w155:dbl)
                n108 = local read "SP_set"() -> (w157:T2)
                n109 = Bundle By Name(cluster=w157, "start(GHz)"=w155, "stop(GHz)"=w154) -> (w158:T2)
                n110 = call "__SET_SP_e4440A.vi"("SP"=w158) -> ()  [unwired: 7 in]
              }
              frame #3 {
                n111 = Wait (ms)(milliseconds to wait=8000) -> ()  [unwired: 1 out]
              }
              frame #4 {
                n112 = GPIB Write(0:w164, 1:":CALC:MARK:MAX") -> (6:w163:errorcluster)  [unwired: 3 in, 1 out]
                n113 = GPIB Write(1:":CALC:MARK:CENT", 3:w163) -> (6:w160:errorcluster)  [unwired: 3 in, 1 out]
                n114 = GPIB Write(1:":FREQ:SPAN 5000;:BAND:res 30Hz", 3:w160) -> ()  [unwired: 3 in, 2 out]
              }
              frame #5 {
                n115 = Wait (ms)(milliseconds to wait=1000) -> ()  [unwired: 1 out]
              }
            }
          }
          frame #4 {
            # "Harmonic IF"
            n116 = local read "Control"() -> (w170:T9)
            n117 = Unbundle By Name(w170) -> ("GPIB_SP"=w169:string)  [unwired: 2 out]
            n118 = flat-sequence {
              tunnel: ":aver:coun 30;:aver on;:aver:cle" -> [w172]
              tunnel: w169 -> [w171]
              tunnel: w169 -> [w176]
              tunnel: [w174] -> w167
              frame #0 {
                n119 = GPIB Write(0:w171, 1:w172) -> ()  [unwired: 3 in, 2 out]
              }
              frame #1 {
                n120 = Wait (ms)(milliseconds to wait=4000) -> ()  [unwired: 1 out]
              }
              frame #2 {
                n121 = call "__SP_mk_peak.vi"("GIPB番号"=w176) -> ("pow out"=w174:dbl, "Freq out"=w175:dbl)  [unwired: 2 in]
                n122 = local write "H IF Pow"(w174) -> ()
                n123 = local write "H IF"(w175) -> ()
              }
            }
          }
          frame #5 {
            n124 = local read "H IF Pow"() -> (w178:dbl)
            n125 = local read "IF Pow"() -> (w177:dbl)
            n126 = local read "H LO"() -> (w183:dbl)
            n127 = local read "H IF"() -> (w182:dbl)
            n128 = local read "LO"() -> (w186:dbl)
            n129 = local read "RF"() -> (w185:dbl)
            n130 = local read "IF"() -> (w184:dbl)
            n131 = Subtract(x=w178, y=w177) -> (x-y=w181:dbl)
            n132 = local read "HLOPopt"() -> (w179:string)
            n133 = local read "LOPopt"() -> (w180:string)
            n134 = Format Into String(format string="%f,%f,%f,%f,  %f,%f,%f,  %f, %s ,%s \\n", initial string=w188, w186, w185, w184, w177, w183, w182, w178, w181, w180, w179) -> (resulting string=w187:string)  [unwired: 1 in, 1 out]
          }
        }
        n135 = Greater Or Equal?(x=w19, y=w32) -> (x >= y?=w31:bool)
        n136 = Insert Into Array(array=w28, new element=w17) -> (w24:dbl[])  [unwired: 1 in]
        n137 = Insert Into Array(array=w30, new element=w19) -> (w25:dbl[])  [unwired: 1 in]
        n138 = Insert Into Array(array=w29, new element=w18) -> (w26:dbl[])  [unwired: 1 in]
        n139 = Bundle(w25, w26) -> (w23:cluster{dbl[], dbl[]})  [unwired: 1 in]
        n140 = Bundle(w25, w24) -> (w22:cluster{dbl[], dbl[]})  [unwired: 1 in]
        n141 = Build Array(w23, w22) -> (→"XYグラフ":cluster{dbl[], dbl[]}[])
        n142 = local write "結果"(w20) -> ()
      }
    }
    frame #2 {
      n143 = local read "LOhharmonic"() -> (w195:T8)
      n144 = local read "Control"() -> (w192:T9)
      n145 = Unbundle By Name(w192) -> ("DATAパス"=w191:path)
      n146 = Unbundle By Name(w195) -> ("save"=w194:bool, "file_name"=w193:string)
      n147 = case shown="참" w194 {
        tunnel: w193 -> [_ w200]
        tunnel: w191 -> [_ w199]
        tunnel: w190 -> [_ w196]
        frame False {
        }
        frame True {
          n148 = Equal?(x=w199, y=path "") -> (x = y?=w201:bool)
          n149 = String Length(string=w200) -> (length=w206:i32)
          n150 = Equal?(x=w206, y=0) -> (x = y?=w202:bool)
          n151 = Or(x=w202, y=w201) -> (x .or. y?=w203:bool)
          n152 = case shown="참" w203 {
            tunnel: w200 -> [w215 _]
            tunnel: [w214 w217] -> w198
            tunnel: [FALSE w216] -> w197
            tunnel: w199 -> [w212 _]
            frame False {
              n153 = Build Path(base path=w212, name or relative path=w215) -> (appended path=w214:path)
            }
            frame True {
              n154 = Open/Create/Replace File(operation (0:open)=5) -> (refnum out=w218:refnum<file>, cancelled=w216:bool)  [unwired: 5 in, 1 out]
              n155 = case shown="거짓" w216 {
                tunnel: w218 -> [w221 _]
                tunnel: [w220 path ""] -> w217
                frame False {
                  n156 = Close File(refnum=w221) -> (path=w220:path)  [unwired: 1 in, 1 out]
                }
                frame True {
                }
              }
            }
          }
          n157 = case shown="참" w197 {
            tunnel: w198 -> [w211 _]
            tunnel: w196 -> [w207 _]
            frame False {
              n158 = Open/Create/Replace File(file path (use dialog)=w211, operation (0:open)=4) -> (refnum out=w209:refnum<file>)  [unwired: 4 in, 2 out]
              n159 = Write to Text File(file (use dialog)=w209, text=w207) -> (refnum out=w208:refnum<file>)  [unwired: 2 in, 2 out]
              n160 = Close File(refnum=w208) -> ()  [unwired: 1 in, 2 out]
            }
            frame True {
            }
          }
        }
      }
    }
  }
